vi "persistence front panel.vi"() -> ()   [LabVIEW 2019]
panel:
  out "Persistence Status":string
  out "Persistent":bool
  in  "Return from persistence":bool
  in  "Make Persistent":bool
  out "Switch Heater\nError":bool
  out "Switch heater \nconfirmed":bool
  out "Switch Heater":bool
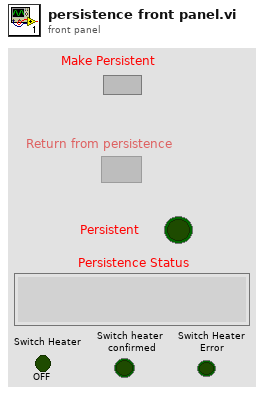
[diagram p1: front panel]
types:
  T1 = enum16{"Always On", "Always Off", "Off While Running"}
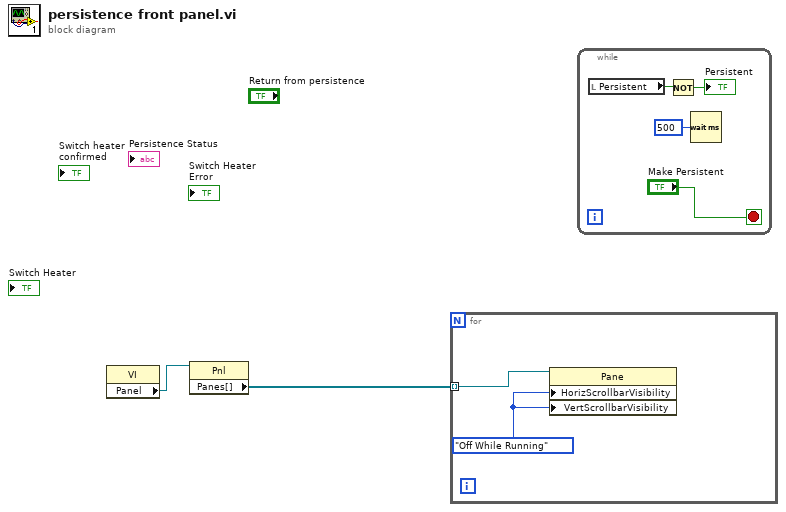
[diagram p0: block diagram]
diagram:
  n1 = property class="VI"() -> ("Panel"=w2:refnum<vi>)  [unwired: 2 in, 2 out]
  n2 = property class="Pnl"(reference=w2) -> ("Panes[]"=w1:refnum<vi>[])  [unwired: 1 in, 2 out]
  n3 = for {
    tunnel: w1 -> [w4] mode=indexing
    w3 = T1."Off While Running" ("Vertical Scrollbar Visibility")
    n4 = property class="Pane"(reference=w4, "HorizScrollbarVisibility"=w3, "VertScrollbarVisibility"=w3) -> ()  [unwired: 1 in, 2 out]
  }
  n5 = while {
    stop <- "Make Persistent" stop-if-true
    n6 = local read "Persistent"() -> (w5:bool)
    n7 = Not(x=w5) -> (.not. x?=→"Persistent":bool)
    n8 = Wait (ms)(milliseconds to wait=u32 500) -> ()  [unwired: 1 out]
  }
